vi "Update Chuck Status.vi"(8 "error in":errorcluster, 10 "Chuck Value":T1, 11 "Chuck Reference In":refnum<vi>) -> (0 "error out":errorcluster)   [LabVIEW 2011]
uses:
  UI typedefs/Chuck Control.ctl
  UI typedefs/Chuck Slot Control.ctl
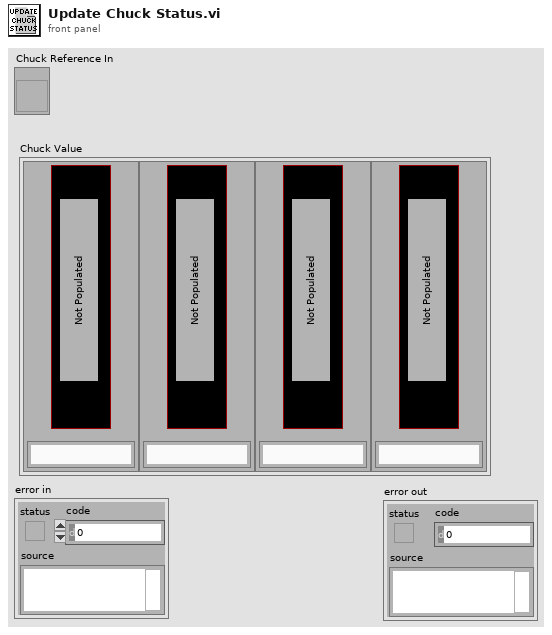
[diagram p1: front panel]
types:
  T1 = typedef "Chuck Control.ctl" = cluster{"Slot 1":T2, "Slot 2":T2, "Slot 3":T2, "Slot 4":T2}
  T2 = typedef "Chuck Slot Control.ctl" = cluster{"Slot Populated":bool, "S/N":string}
  T3 = enum8{"Enabled", "Disabled", "Disabled and Grayed Out"}
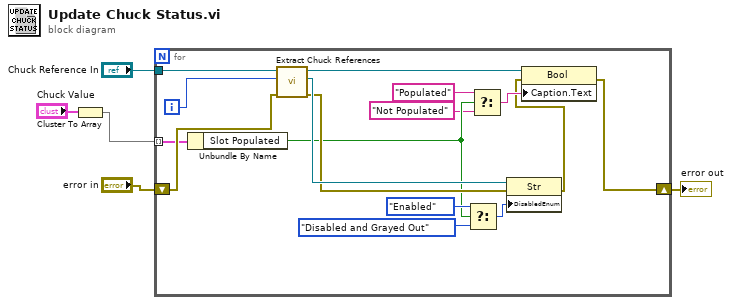
[diagram p0: block diagram]
diagram:
  n1 = Cluster To Array(cluster="Chuck Value") -> (array=w2:T2[])
  n2 = for {
    tunnel: "Chuck Reference In" -> [w21]
    tunnel: w2 -> [w18] mode=indexing
    shift-right: [w6] -> w1
    shift-left: "error in" -> [w20]
    i -> [w19]
    n3 = Unbundle By Name(w18) -> ("Slot Populated"=w10:bool)
    n4 = call "Extract Chuck References.vi"("error in"=w20, "Slot"=w19, "Chuck Reference"=w21) -> ("error out"=w16:errorcluster, "Serial Number Reference"=w17:refnum<vi>, "Populated Button Reference"=w12:refnum<vi>)  [unwired: 6 in]
    n5 = Select(t=T3."Enabled" ("Disabled"), s=w10, f=T3."Disabled and Grayed Out" ("Disabled")) -> (s? t:f=w14:T3)
    n6 = Select(t="Populated", s=w10, f="Not Populated") -> (s? t:f=w11:string)
    n7 = property class="Str"(reference=w17, error in=w16, "DisabledEnum"=w14) -> (error out=w7:errorcluster)  [unwired: 1 out]
    n8 = property class="Bool"(reference=w12, error in=w7, "Caption.Text"=w11) -> (error out=w6:errorcluster)  [unwired: 1 out]
  }
  "error out" <- w1
